vi "SpectrometerSMO.vi"() -> ()   [LabVIEW 2017]
doc: "Use this template to build a VI to use as a subVI."
uses:
  Spectrometer Utilities/SpectrometerData.ctl
  Spectrometer Utilities/SpectrometerCallbackdataEvent.ctl
  <vilib>/Utility/config.llb/Write Key (I32).vi
  <vilib>/Utility/config.llb/Write Key (String).vi
  <vilib>/Utility/config.llb/Read Key (I32).vi
  <vilib>/Utility/config.llb/NI_LVConfig.lvlib
panel:
  in  "user event Callback":refnum<user-event>
  out "Spectrometer Data Ouput":T1
  out "Grating 2":string="1800 gr/mm" caption="String"
  in  "Grating":string="Grating" caption="String"
  out "Accumulations 2":string="3" caption="String"
  out "Range 2":string="21531...16531 abs cm-¹" caption="String"
  out "Binning 2":string="1" caption="String"
  out "Laser 2":string="512 nm" caption="String"
  out "Slit 2":string="150.0010 µm" caption="String"
  out "Hole 2":string="70.0087 µm" caption="String"
  out "Windows 2":string="3" caption="String"
  out "Acquired Time 2":string="18.10.2017 15:05:12" caption="String"
  out "Acq Time 2":string="0.154 s" caption="String"
  in  "Acquired Time":string="Date and time" caption="String"
  in  "Windows":string="Windows" caption="String"
  in  "Hole":string="Hole" caption="String"
  in  "Slit":string="Slit" caption="String"
  in  "Laser":string="Laser" caption="String"
  in  "Binning":string="Binning" caption="String"
  in  "Range":string="Range" caption="String"
  in  "Accumulations":string="Accumulations" caption="String"
  in  "Acq Time":string="Acq. Time" caption="String"
  out "Raman Spectra from FHR":cluster{"Array":dbl[], "Array":dbl[]}(graph) caption="XY Graph - dark"
  in  "BasePath":path=path "C:/Users/OmerLab/Documents/GitHub/RamanSpecUsingStageXY" caption="Path"
  in  "CommandFileName":string="SpectrometerCommand.txt" caption="String"
  in  "StatusFileName":string="SpectrometerStatus.txt" caption="String"
  in  "SavedSpectrumFileName":string="DateTimeSpectrumPointNumber1.txt" caption="String"
  out "MeasurementStringView":string="Spectrometer" caption="String"
  out "MeasurementInProgressView":bool
  in  "SpectrometerString":string="Spectrometer" caption="String"
  in  "StageString":string="Stage" caption="String"
  out "Stage":bool
  in  "CameraString":string="Camera" caption="String"
  out "Camera":bool
  in  "SpectrometerString":string="Spectrometer" caption="String"
  out "SpectrometerView":bool=TRUE
  in  "Numeric":dbl
  in  "Close":bool=TRUE
  in  "Abort":bool
  in  "Pause":bool
  in  "Stop":bool
  in  "RequestSpectrometer2StartMeasurement":bool caption="Start"
  in  "Help":bool
  in  "User":bool
  out "TimeStampView":timestamp=timestamp(3591173163 s since 1904-01-01) format="%<%.0X %x>T"
  out "error out 2":errorcluster {"code" format="Error %.0f"}
  in  "error in (no error) 2":errorcluster {"code" format="Error %.0f"}
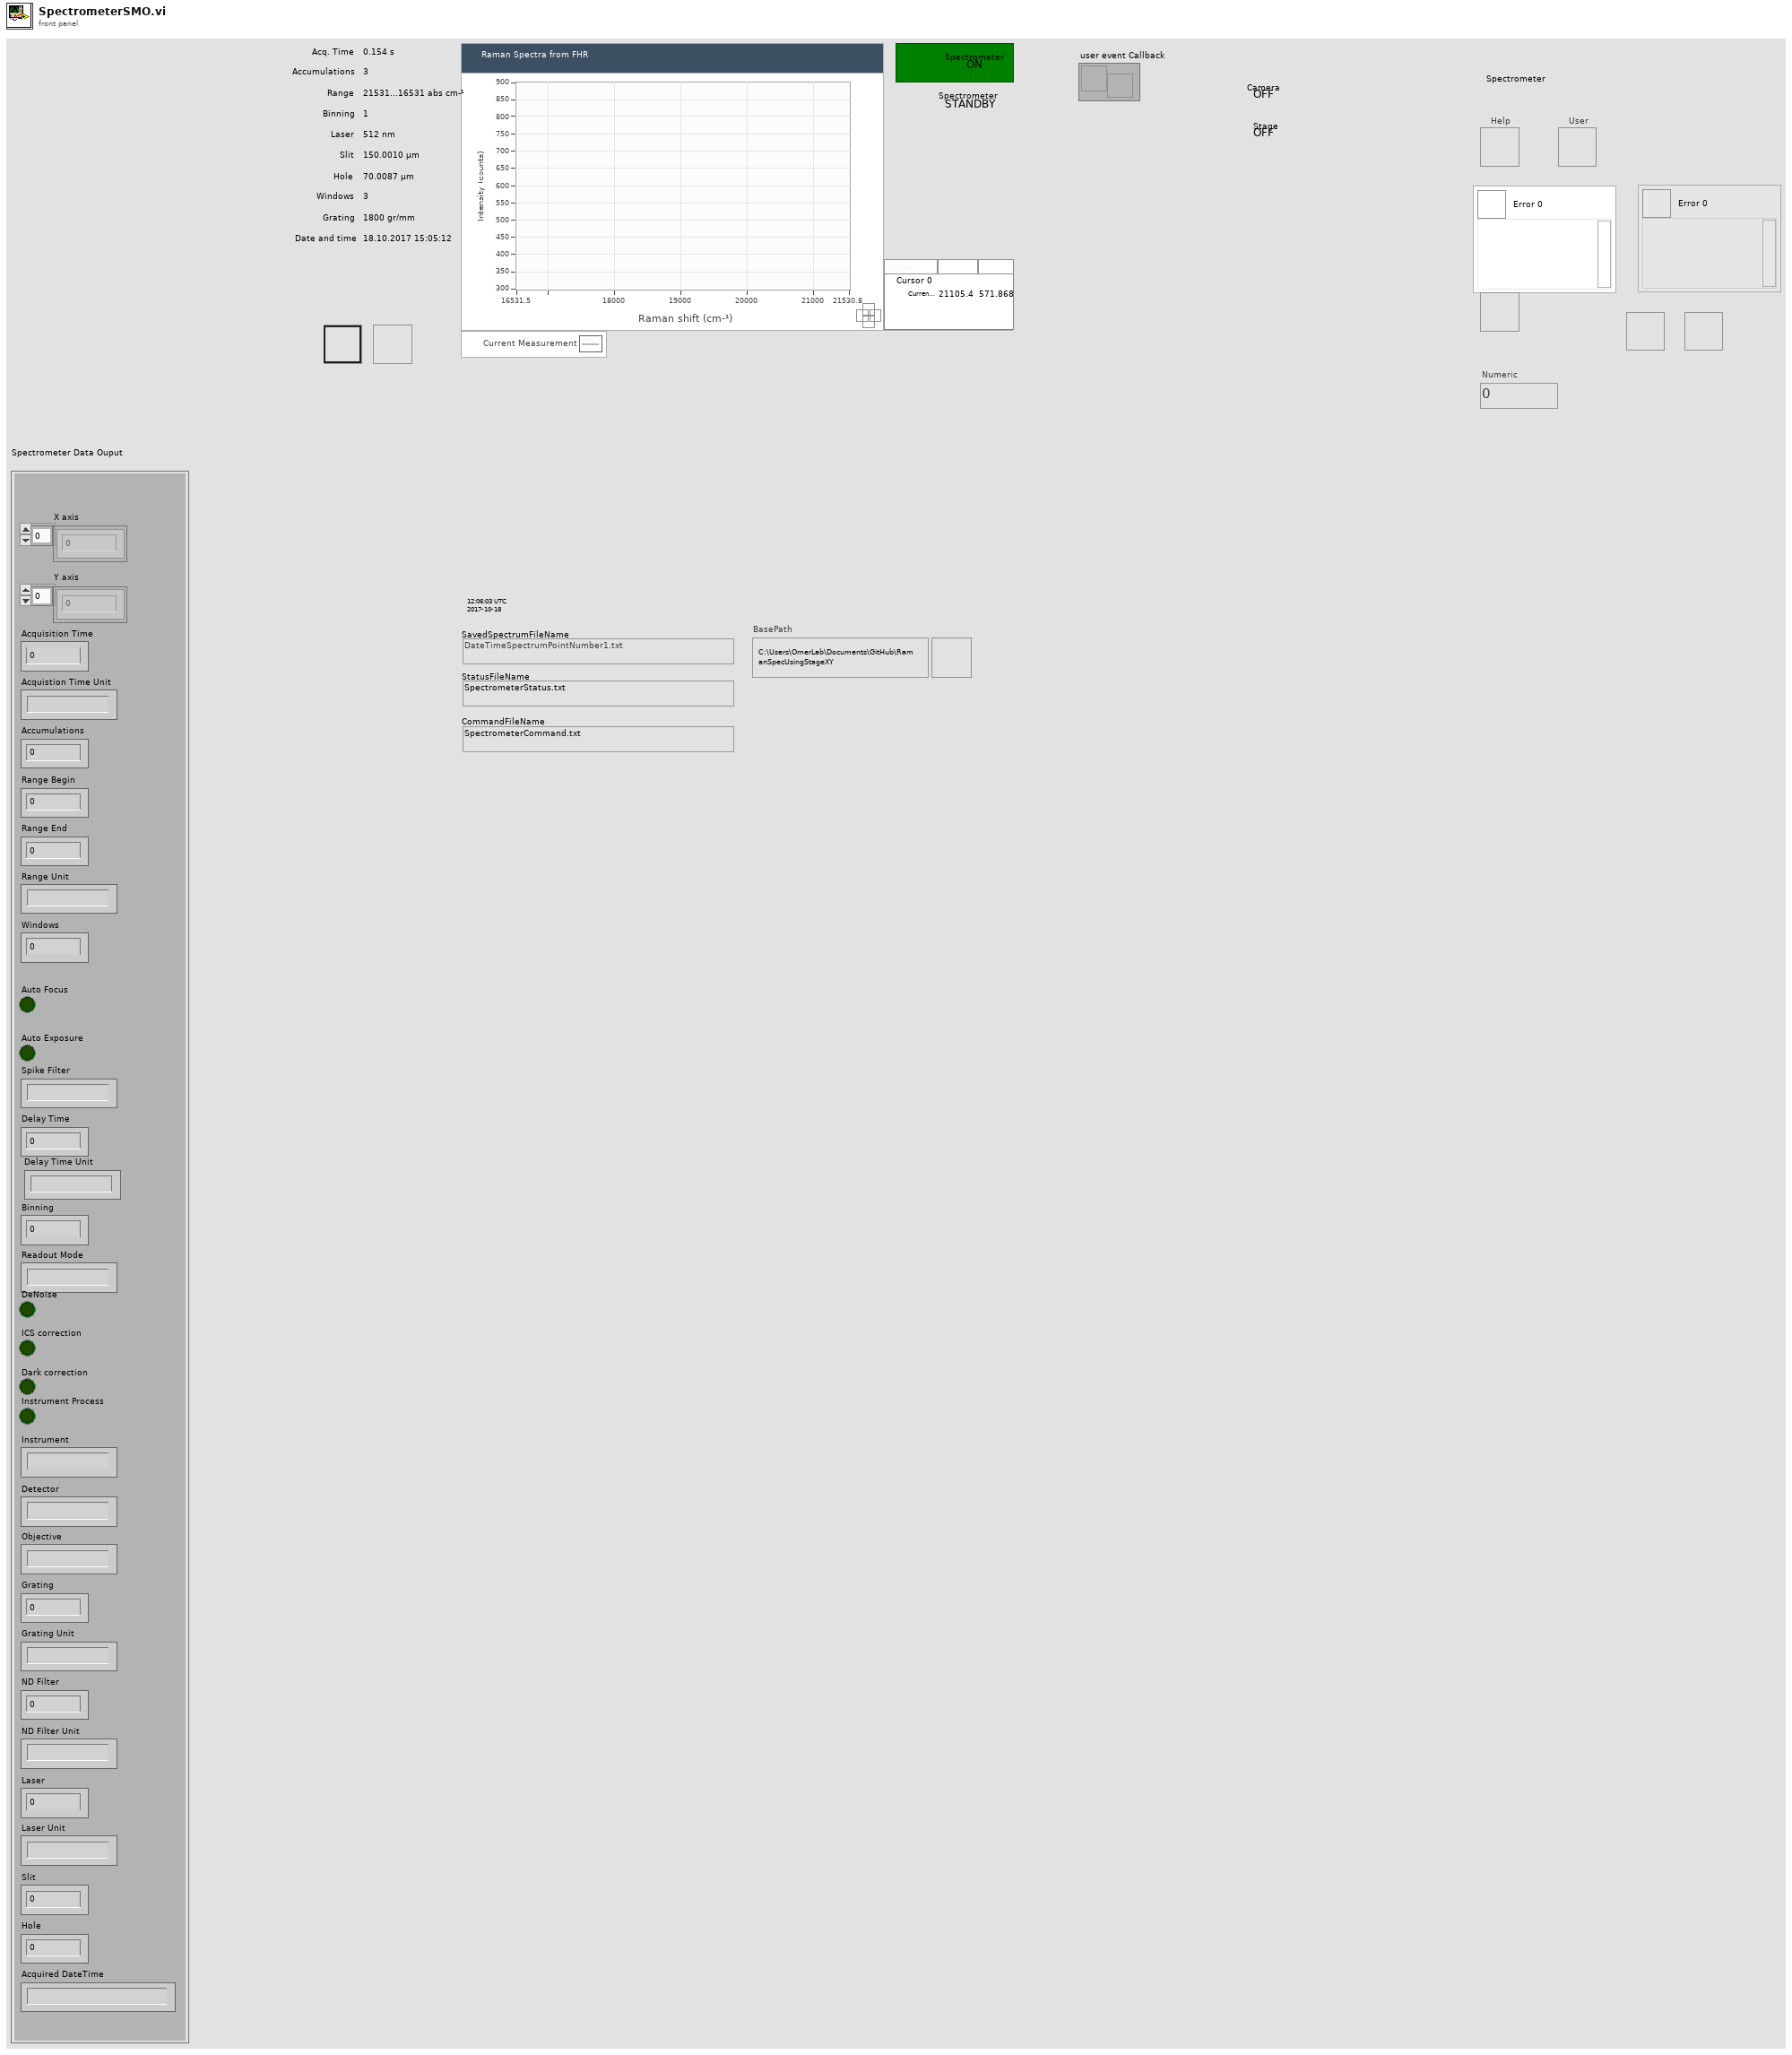
[diagram p1: front panel]
types:
  T1 = typedef "SpectrometerData.ctl" = cluster{"Acquisition Time":dbl, "Range Begin":dbl, "Acquistion Time Unit":string, "Accumulations":i32, "Range End":dbl, "Range Unit":string, "Windows":i32, "Auto Focus":bool, "Auto Exposure":bool, "Spike Filter":string, "Delay Time":dbl, "Delay Time Unit":string, "Binning":i32, "Readout Mode":string, "DeNoise":bool, "ICS correction":bool, "Dark correction":bool, "Instrument Process":bool, "Instrument":string, "Detector":string, "Objective":string, "Grating":i32, "Grating Unit":string, "ND Filter":dbl, "ND Filter Unit":string, "Laser":dbl, "Laser Unit":string, "Slit":dbl, "Hole":dbl, "Acquired DateTime":string, "X axis":dbl[], "Y axis":dbl[]}
  T2 = typedef "SpectrometerCallbackdataEvent.ctl" = cluster{"MeasurementEndedSuccessfully?":bool, "Spectrometer Connected?":bool, "Measurement In Progress?":bool}
  T3 = typedef "NI_LVConfig.lvlib/Config Data RefNum.ctl" = refnum<k1>
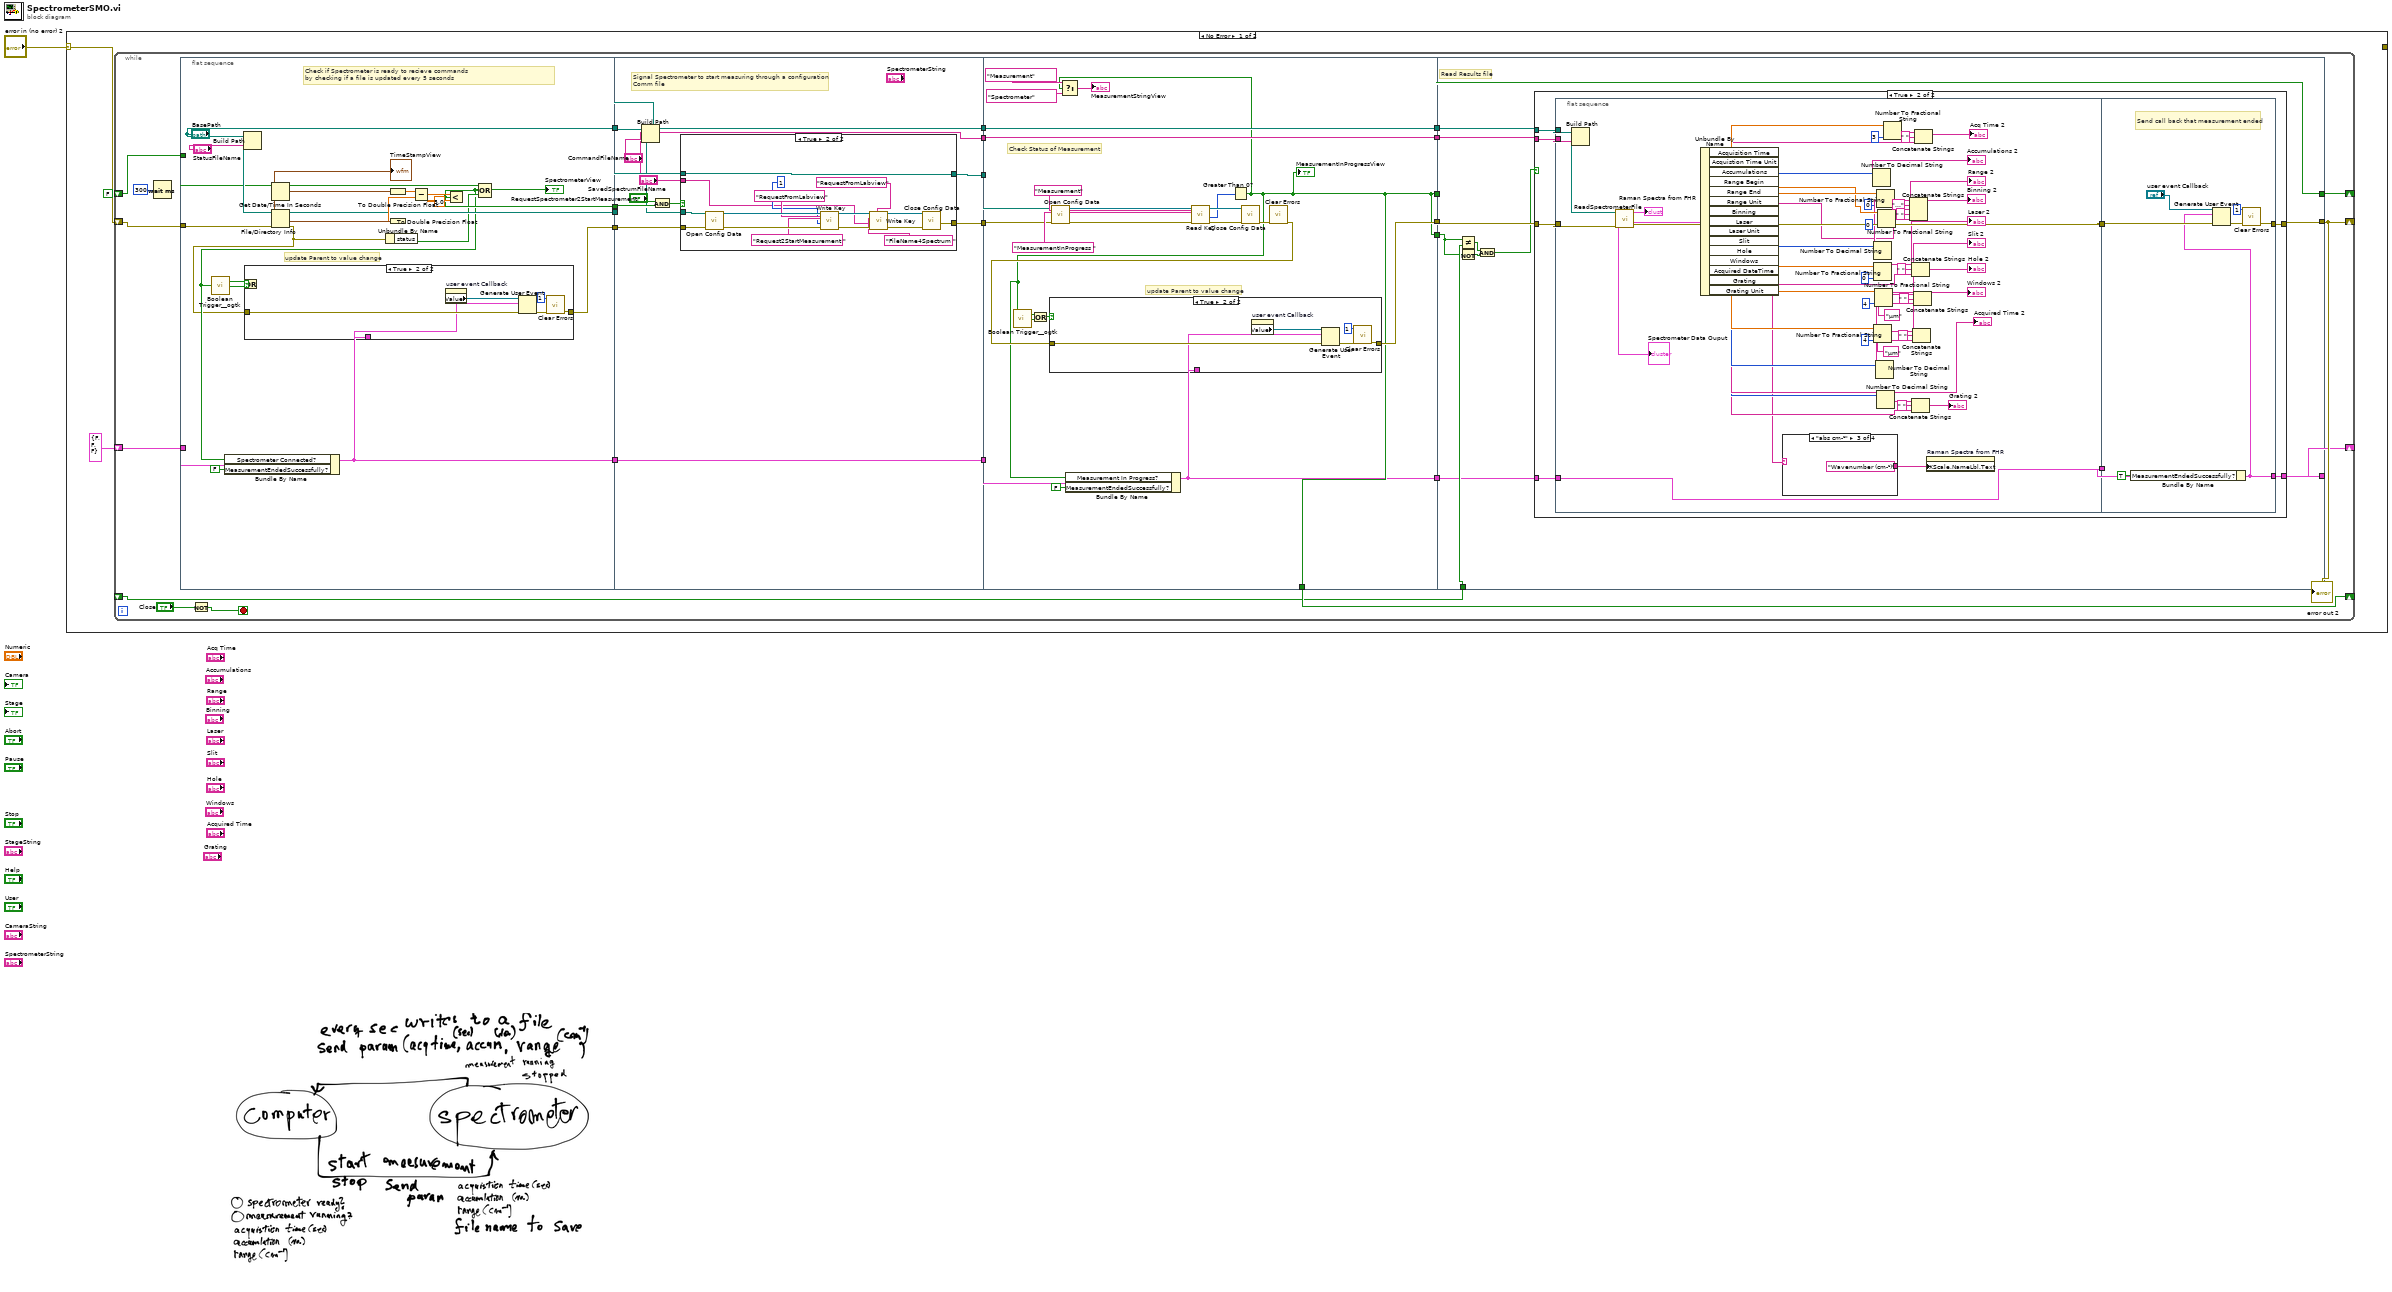
[diagram p0: block diagram]
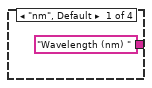
[diagram p6: hidden frame]
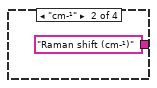
[diagram p7: hidden frame]
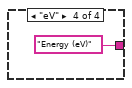
[diagram p8: hidden frame]
diagram:
  n1 = case shown="No Error" "error in (no error) 2" {
    selector: "error in (no error) 2" -> [w4 w212]
    tunnel: [_ w212] -> _
    frame No Error {
      n2 = while {
        shift-right: [w22] -> _
        shift-left: w4 -> [w30]
        shift-right: [w24] -> _
        shift-left: FALSE -> [w23]
        shift-right: [w14] -> _
        shift-left: _ -> [w13]
        shift-right: [w5] -> _
        shift-left: T2 {"MeasurementEndedSuccessfully?"=FALSE, "Spectrometer Connected?"=FALSE, "Measurement In Progress?"=FALSE} ("event data") -> [w9]
        stop <- w10 stop-if-true
        n3 = Wait (ms)(milliseconds to wait=u32 300) -> ()  [unwired: 1 out]
        n4 = flat-sequence {
          tunnel: w30 -> [w48]
          tunnel: [w37] -> w29
          tunnel: [w47] -> w28
          tunnel: [w42] -> w27
          tunnel: w23 -> [w43]
          tunnel: ["BasePath"] -> w19
          tunnel: w9 -> [w36]
          tunnel: [w34] -> w8
          tunnel: w29 -> [w73]
          tunnel: w28 -> [w68]
          tunnel: w27 -> [w70]
          tunnel: [w72] -> w26
          tunnel: [w67] -> w25
          tunnel: w19 -> [w63]
          tunnel: ["SavedSpectrumFileName"] -> w17
          tunnel: [w63] -> w15
          tunnel: w8 -> [w62]
          tunnel: [w62] -> w7
          tunnel: w26 -> [w109]
          tunnel: w25 -> [w108]
          tunnel: [w96] -> w21
          tunnel: [w94] -> w20
          tunnel: [w102] -> w18
          tunnel: w17 -> [w102]
          tunnel: [w101] -> w16
          tunnel: w15 -> [w101]
          tunnel: [w94] -> w14
          tunnel: [w94] -> w12
          tunnel: w7 -> [w95]
          tunnel: [w93] -> w6
          tunnel: [w134] -> w24
          tunnel: [w130] -> w22
          tunnel: w21 -> [w131]
          tunnel: w20 -> [w134]
          tunnel: w18 -> [w132]
          tunnel: w16 -> [w133]
          tunnel: w13 -> [w129]
          tunnel: w12 -> [w128]
          tunnel: w6 -> [w124]
          tunnel: [w123] -> w5
          frame #0 {
            # "update Parent to value change"
            # "Check if Spectrometer is ready to recieve commands\nby checking if a file is updated every 5 seconds"
            n5 = Build Path(base path="BasePath", name or relative path="StatusFileName") -> (appended path=w45:path)
            n6 = Get Date/Time In Seconds() -> (seconds since 1Jan1904=w53:timestamp)
            n7 = File/Directory Info(path=w45, error in=w48) -> (path out=w47:path, last mod=w54:timestamp, error out=w32:errorcluster)  [unwired: 4 out]
            "TimeStampView" <- w54
            n8 = Unbundle By Name(w32) -> ("status"=w41:bool)
            n9 = To Double Precision Float(number=w53) -> (double precision float=w52:dbl)
            n10 = To Double Precision Float(number=w54) -> (double precision float=w51:dbl)
            n11 = Subtract(x=w52, y=w51) -> (x-y=w50:dbl)
            n12 = Less?(x=w50, y=5.0) -> (x < y?=w42:bool)
            n13 = Compound Arithmetic op=OR(w43, w42, w41) -> (w35:bool)
            "SpectrometerView" <- w35
            n14 = call <userlib>:"Boolean Trigger__ogtk.vi"("Boolean Input"=w35) -> ("Rising Edge"=w40:bool, "Falling Edge"=w39:bool)  [unwired: 1 in]
            n15 = Bundle By Name(cluster=w36, "Spectrometer Connected?"=w35, "MeasurementEndedSuccessfully?"=FALSE) -> (w34:T2)
            n16 = Or(x=w40, y=w39) -> (x .or. y?=w38:bool)
            n17 = case shown="True" w38 {
              tunnel: [w55 w57] -> w37
              tunnel: w32 -> [w55 w60]
              tunnel: w34 -> [_ w59]
              frame False {
              }
              frame True {
                n18 = property on="user event Callback" class="TypRef (strict)"() -> ("Value"=w61:refnum<user-event>)  [unwired: 2 in, 2 out]
                n19 = Generate User Event(user event=w61, event data cluster=w59, error in=w60) -> (error out=w58:errorcluster)  [unwired: 1 in, 1 out]
                n20 = call <vilib>:"Clear Errors.vi"("error in (no error)"=w58, "specific error code to clear (0: all)"=1) -> ("error out"=w57:errorcluster)  [unwired: 4 in, 1 out]
              }
            }
          }
          frame #1 {
            # "Signal Spectrometer to start measuring through a configuration\nComm file"
            n21 = Build Path(base path=w63, name or relative path="CommandFileName") -> (appended path=w65:path)
            n22 = And(x="RequestSpectrometer2StartMeasurement", y=w70) -> (x .and. y?=w69:bool)
            n23 = case shown="True" w69 {
              tunnel: w73 -> [w75 w90]
              tunnel: w65 -> [_ w89]
              tunnel: [w75 w85] -> w72
              tunnel: w68 -> [w74 w83]
              tunnel: [w74 w83] -> w67
              tunnel: "SavedSpectrumFileName" -> [_ w76]
              frame False {
              }
              frame True {
                n24 = call <vilib>:"Open Config Data.vi"("error in (no error)"=w90, "configuration file path"=w89) -> ("error out"=w91:errorcluster, "refnum"=w88:T3)  [unwired: 7 in, 1 out]
                n25 = call-poly <vilib>:"Write Key.vi"("section"="RequestFromLabview", "error in (no error)"=w91, "value"=1, "key"="Request2StartMeasurement ", "refnum"=w88) -> ("error out"=w79:errorcluster, "refnum out"=w82:T3)  [unwired: 4 in, 1 out]
                n26 = call-poly <vilib>:"Write Key.vi"("section"="RequestFromLabview", "error in (no error)"=w79, "value"=w76, "key"="FileName4Spectrum ", "refnum"=w82) -> ("error out"=w80:errorcluster, "refnum out"=w81:T3)  [unwired: 4 in, 1 out]
                n27 = call <vilib>:"Close Config Data.vi"("error in (no error)"=w80, "refnum"=w81) -> ("error out"=w85:errorcluster)  [unwired: 8 in, 1 out]
              }
            }
          }
          frame #2 {
            # "update Parent to value change"
            # "Check Status of Measurement"
            n28 = call <vilib>:"Open Config Data.vi"("error in (no error)"=w109, "configuration file path"=w108) -> ("error out"=w110:errorcluster, "refnum"=w112:T3)  [unwired: 7 in, 1 out]
            n29 = call-poly <vilib>:"Read Key.vi"("section"="Measurement", "error in (no error)"=w110, "key"="MeasurementInProgress ", "refnum"=w112) -> ("error out"=w111:errorcluster, "value"=w107:i32, "refnum out"=w115:T3)  [unwired: 4 in, 1 out]
            n30 = Greater Than 0?(x=w107) -> (x > 0?=w94:bool)
            "MeasurementInProgressView" <- w94
            n31 = call <userlib>:"Boolean Trigger__ogtk.vi"("Boolean Input"=w94) -> ("Rising Edge"=w98:bool, "Falling Edge"=w99:bool)  [unwired: 1 in]
            n32 = Or(x=w98, y=w99) -> (x .or. y?=w100:bool)
            n33 = Select(t="Measurement" ("section"), s=w94, f="Spectrometer" ("section")) -> (s? t:f=→"MeasurementStringView":string)
            n34 = Bundle By Name(cluster=w95, "Measurement In Progress?"=w94, "MeasurementEndedSuccessfully?"=FALSE) -> (w93:T2)
            n35 = call <vilib>:"Close Config Data.vi"("error in (no error)"=w111, "refnum"=w115) -> ("error out"=w106:errorcluster)  [unwired: 8 in, 1 out]
            n36 = call <vilib>:"Clear Errors.vi"("error in (no error)"=w106) -> ("error out"=w97:errorcluster)  [unwired: 5 in, 1 out]
            n37 = case shown="True" w100 {
              tunnel: [w116 w117] -> w96
              tunnel: w97 -> [w116 w121]
              tunnel: w93 -> [_ w120]
              frame False {
              }
              frame True {
                n38 = property on="user event Callback" class="TypRef (strict)"() -> ("Value"=w122:refnum<user-event>)  [unwired: 2 in, 2 out]
                n39 = Generate User Event(user event=w122, event data cluster=w120, error in=w121) -> (error out=w118:errorcluster)  [unwired: 1 in, 1 out]
                n40 = call <vilib>:"Clear Errors.vi"("error in (no error)"=w118, "specific error code to clear (0: all)"=1) -> ("error out"=w117:errorcluster)  [unwired: 4 in, 1 out]
              }
            }
          }
          frame #3 {
            # "Read Results file"
            n41 = Not Equal?(x=w128, y=w129) -> (x != y?=w126:bool)
            n42 = Not(x=w128) -> (.not. x?=w127:bool)
            n43 = And(x=w126, y=w127) -> (x .and. y?=w125:bool)
            n44 = case shown="True" w125 {
              tunnel: w133 -> [_ w144]
              tunnel: w132 -> [_ w143]
              tunnel: w131 -> [w136 w142]
              tunnel: [w136 w141] -> w130
              tunnel: w124 -> [w135 w138]
              tunnel: [w135 w137] -> w123
              frame False {
              }
              frame True {
                n45 = flat-sequence {
                  tunnel: w144 -> [w199]
                  tunnel: w143 -> [w198]
                  tunnel: w142 -> [w196]
                  tunnel: [w195] -> w140
                  tunnel: [w145] -> w139
                  tunnel: w138 -> [w145]
                  tunnel: [w204] -> w141
                  tunnel: w140 -> [w210]
                  tunnel: w139 -> [w209]
                  tunnel: [w207] -> w137
                  frame #0 {
                    n46 = Build Path(base path=w199, name or relative path=w198) -> (appended path=w197:path)
                    n47 = call "ReadSpectrometerFile.vi"("error in (no error)"=w196, "FileNameAndPath"=w197) -> ("error out"=w195:errorcluster, "Spectrometer Data Ouput"=w193:T1, "Spectrometer Result"=→"Raman Spectra from FHR":cluster{"Array":dbl[], "Array":dbl[]})  [unwired: 7 in]
                    "Spectrometer Data Ouput" <- w193
                    n48 = Unbundle By Name(w193) -> ("Acquisition Time"=w192:dbl, "Acquistion Time Unit"=w189:string, "Accumulations"=w187:i32, "Range Begin"=w185:dbl, "Range End"=w183:dbl, "Range Unit"=w147:string, "Binning"=w178:i32, "Laser"=w176:dbl, "Laser Unit"=w173:string, "Slit"=w171:dbl, "Hole"=w163:dbl, "Windows"=w161:i32, "Acquired DateTime"=→"Acquired Time 2":string, "Grating"=w152:i32, "Grating Unit"=w149:string)
                    n49 = case shown="\"abs cm-¹\"" w147 {
                      tunnel: ["Wavelength (nm) " ("string") "Raman shift (cm-¹)" ("string") "Wavenumber (cm-¹)" ("string") "Energy (eV)" ("string")] -> w146
                      frame "nm", Default {
                      }
                      frame "cm-¹" {
                      }
                      frame "abs cm-¹" {
                      }
                      frame "eV" {
                      }
                    }
                    n50 = Number To Decimal String(number=w187) -> (decimal integer string=→"Accumulations 2":string)  [unwired: 1 in]
                    n51 = Number To Fractional String(number=w176, precision (6)=i16 0) -> (F-format string=w175:string)  [unwired: 2 in]
                    n52 = Number To Decimal String(number=w178) -> (decimal integer string=→"Binning 2":string)  [unwired: 1 in]
                    n53 = Number To Fractional String(number=w163, precision (6)=i16 4) -> (F-format string=w164:string)  [unwired: 2 in]
                    n54 = Number To Fractional String(number=w171, precision (6)=i16 4) -> (F-format string=w170:string)  [unwired: 2 in]
                    n55 = Number To Decimal String(number=w161) -> (decimal integer string=→"Windows 2":string)  [unwired: 1 in]
                    n56 = Number To Fractional String(number=w185, precision (6)=i16 0) -> (F-format string=w182:string)  [unwired: 2 in]
                    n57 = Number To Decimal String(number=w152) -> (decimal integer string=w151:string)  [unwired: 1 in]
                    n58 = Number To Fractional String(number=w183, precision (6)=i16 0) -> (F-format string=w184:string)  [unwired: 2 in]
                    n59 = Number To Fractional String(number=w192, precision (6)=i16 3) -> (F-format string=w191:string)  [unwired: 2 in]
                    n60 = Concatenate Strings(w182, "..." ("string"), w184, " " ("string"), w147) -> (→"Range 2":string)
                    n61 = Concatenate Strings(w175, " " ("string"), w173) -> (→"Laser 2":string)
                    n62 = Concatenate Strings(w151, " " ("string"), w149) -> (→"Grating 2":string)
                    n63 = Concatenate Strings(w164, " " ("string"), "µm" ("string")) -> (→"Hole 2":string)
                    n64 = Concatenate Strings(w170, " " ("string"), "µm" ("string")) -> (→"Slit 2":string)
                    n65 = Concatenate Strings(w191, " " ("string"), w189) -> (→"Acq Time 2":string)
                    n66 = property on="Raman Spectra from FHR" class="XYGraph (strict)"("XScale.NameLbl.Text"=w146) -> ()  [unwired: 2 in, 2 out]
                  }
                  frame #1 {
                    # "Send call back that measurement ended"
                    n67 = Bundle By Name(cluster=w209, "MeasurementEndedSuccessfully?"=TRUE) -> (w207:T2)
                    n68 = Generate User Event(user event="user event Callback", event data cluster=w207, error in=w210) -> (error out=w205:errorcluster)  [unwired: 1 in, 1 out]
                    n69 = call <vilib>:"Clear Errors.vi"("error in (no error)"=w205, "specific error code to clear (0: all)"=1) -> ("error out"=w204:errorcluster)  [unwired: 4 in, 1 out]
                  }
                }
              }
            }
          }
        }
        n70 = Not(x="Close") -> (.not. x?=w10:bool)
        "error out 2" <- w22
      }
    }
    frame Error {
    }
  }
